vi "NXTUnspecifiedString.vi"() -> (1 "NXT Target: Unspecified String":string="NXT Target: Unspecified")   [LabVIEW 2010]
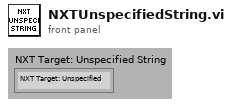
[diagram p1: front panel]
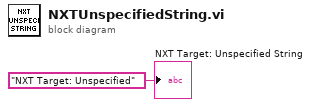
[diagram p0: block diagram]
diagram:
  "NXT Target: Unspecified String" <- "NXT Target: Unspecified" ("String")
